vi "AWS-S3-PutObjectData.vi"(0 "AWS-S3-API":refnum<class "AWS-S3-API.lvclass">, 1 "Headers":T1[](array[typedef])=[{"Key"="Content-Type", "Value"="application/octet-stream"}], 2 "Timeout (3600000msec=1hr)":i32=3600000 format="%dmsec", 5 "Object Key":string, 7 "Object Bucket":string, 9 "Object Data":string, 11 "error in":errorcluster, 12 "Metadata":T1[](array[typedef]), 13 "ReadWriteTimeout (3600000msec=1hr)":i32=3600000 format="%dmsec") -> (4 "AWS-S3-API out":refnum<class "AWS-S3-API.lvclass">, 6 "ResponseXml":string, 8 "Object URL":string, 15 "error out":errorcluster)   [LabVIEW 2012, in "AWS-S3-API.lvclass"]
uses:
  AWS-S3-API.lvclass
  C:/Users/Jack/repo/aws/AWS-SDK/AWSSDK.dll
  repo/aws/AWS-SDK/AWSSDK.dll
  AWS Shared/AWS-Shared-MetadataKeyValuePair.ctl
panel:
  # "Inputs"
  # "Outputs"
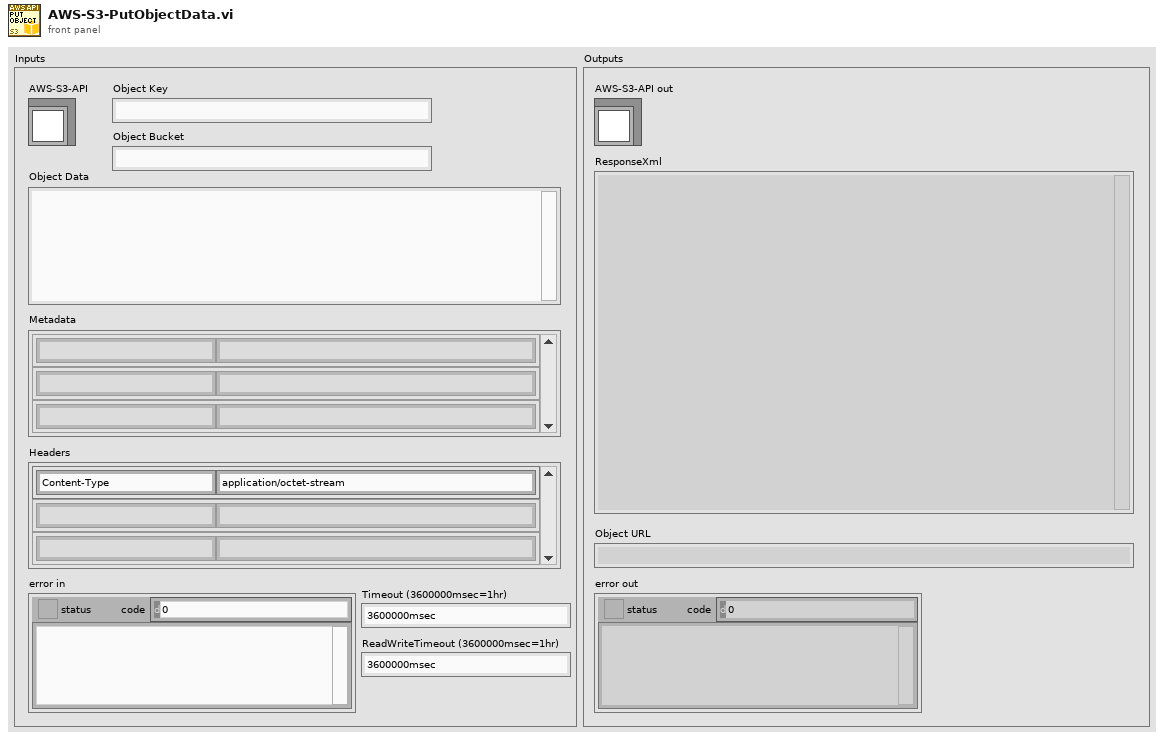
[diagram p1: front panel]
types:
  T1 = typedef "AWS-Shared-MetadataKeyValuePair.ctl" = cluster{"Key":string, "Value":string}
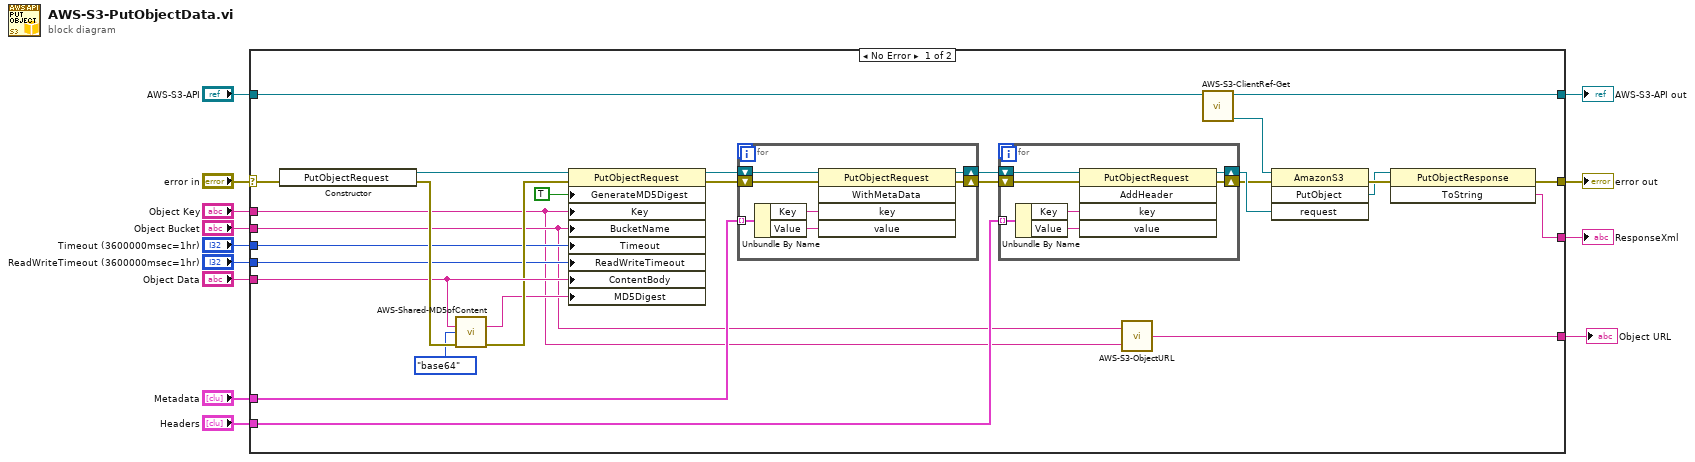
[diagram p0: block diagram]
diagram:
  n1 = case shown="No Error" "error in" {
    selector: "error in" -> [w40 w57]
    tunnel: [w35 w57] -> w13
    tunnel: [w23 w56] -> w11
    tunnel: "AWS-S3-API" -> [w24 w56]
    tunnel: "Object Data" -> [w26 _]
    tunnel: "Object Key" -> [w15 _]
    tunnel: "Object Bucket" -> [w16 _]
    tunnel: "Metadata" -> [w38 _]
    tunnel: [w34 _] -> w5
    tunnel: "Headers" -> [w31 _]
    tunnel: "Timeout (3600000msec=1hr)" -> [w18 _]
    tunnel: "ReadWriteTimeout (3600000msec=1hr)" -> [w17 _]
    tunnel: [w14 _] -> w1
    frame No Error {
      n2 = constructor class="PutObjectRequest"(error in=w40) -> (reference out=w39:refnum<k24>, error out=w41:errorcluster)  [unwired: 2 in, 1 out]
      n3 = call "AWS-Shared-MD5ofContent.vi"("Content"=w26, "Encoding"=enum16{"base64", "ASCII Hex"}."base64", "error in"=w41) -> ("MD5"=w19:string, "error out"=w20:errorcluster)  [unwired: 11 in]
      n4 = property class="PutObjectRequest"(reference=w39, error in=w20, "GenerateMD5Digest"=TRUE, "Key"=w15, "BucketName"=w16, "Timeout"=w18, "ReadWriteTimeout"=w17, "ContentBody"=w26, "MD5Digest"=w19) -> (reference out=w28:refnum<k24>, error out=w27:errorcluster)
      n5 = for {
        shift-right: [w52] -> w30
        shift-left: w28 -> [w55]
        shift-right: [w53] -> w32
        shift-left: w27 -> [w54]
        tunnel: w38 -> [w51] mode=indexing
        n6 = Unbundle By Name(w51) -> ("Key"=w50:string, "Value"=w49:string)
        n7 = invoke class="PutObjectRequest" method="WithMetaData"(reference=w55, error in=w54, "key"=w50, "value"=w49) -> (reference out=w52:refnum<k24>, error out=w53:errorcluster)  [unwired: 1 in, 3 out]
      }
      n8 = for {
        shift-right: [w45] -> w29
        shift-left: w30 -> [w48]
        shift-right: [w46] -> w22
        shift-left: w32 -> [w47]
        tunnel: w31 -> [w44] mode=indexing
        n9 = Unbundle By Name(w44) -> ("Key"=w43:string, "Value"=w42:string)
        n10 = invoke class="PutObjectRequest" method="AddHeader"(reference=w48, error in=w47, "key"=w43, "value"=w42) -> (reference out=w45:refnum<k24>, error out=w46:errorcluster)  [unwired: 1 in, 3 out]
      }
      n11 = call "AWS-S3-ObjectURL.vi"("Object Bucket"=w16, "Object Key"=w15) -> ("Object URL"=w14:string)  [unwired: 2 in]
      n12 = call "AWS-S3-ClientRef-Get.vi"("AWS-S3-API"=w24) -> ("S3 Client ref"=w25:refnum<k24>, "AWS-S3-API out"=w23:refnum<class "AWS-S3-API.lvclass">)  [unwired: 9 in]
      n13 = invoke class="AmazonS3" method="PutObject"(reference=w25, error in=w22, "request"=w29) -> (error out=w36:errorcluster, "PutObject"=w33:refnum<k24>)  [unwired: 1 in, 2 out]
      n14 = invoke class="PutObjectResponse" method="ToString"(reference=w33, error in=w36) -> (error out=w35:errorcluster, "ToString"=w34:string)  [unwired: 1 in, 1 out]
    }
    frame Error {
    }
  }
  "error out" <- w13
  "AWS-S3-API out" <- w11
  "ResponseXml" <- w5
  "Object URL" <- w1
